vi "Top_Level.vi"() -> ()   [LabVIEW 2013]
uses:
  Classes/OSSP_Problem.lvclass
  Classes/GA.lvclass
  Classes/GA_Class/Controls/Solution.ctl
  Classes/GA_Class/Controls/Strategy.ctl
  Controls/States.ctl
  Classes/GA.lvclass/GA.ctl
  Classes/GA_Class/Evaluate Single Solution.vi
  Classes/GA_Class/Calculate Makespan.vi
  Classes/GA_Class/Select Random Solutions_2.vi
  Classes/GA_Class/One Point Crossover.vi
  Classes/Find Best Solution In Population.vi
  Classes/GA_Class/GA_Operation_To_MachineJobTuple.vi
  Classes/GA_Class/Find Gaps On Particular Machine.vi
  Classes/GA_Class/GA_Check_Other_Machines.vi
  Classes/GA_Class/GA_Schedule_Job.vi
  Classes/GA_Class/GA_Find_Job_On_Other_Machines.vi
  Classes/GA_Class/Find Elements not On Other Child.vi
  <vilib>/Analysis/baseanly.llb/Mean.vi
  <vilib>/Analysis/baseanly.llb/Mean (DBL).vi
  <vilib>/Analysis/1siggen.llb/Riffle.vi
  <vilib>/Analysis/1siggen.llb/Riffle Array (I32).vi
  Classes/GA_Class/GA_Increment_NumberofJobsOn Machine_ByOne.vi
panel:
  in  "Strategy":T1
  in  "Number of Generations":i32=1000
  in  "Population Size":u8=80
  in  "Mutation Probability":dbl=0.2
  in  "Crossover Probability":dbl=0.75
  out "Picture":picture
  out "Best Solution":T2
  out "GA.lvclass":refnum<class "GA.lvclass">
  out "OSSP_Problem.lvclass":refnum<class "OSSP_Problem.lvclass">
  out "error out":errorcluster
  in  "error in":errorcluster
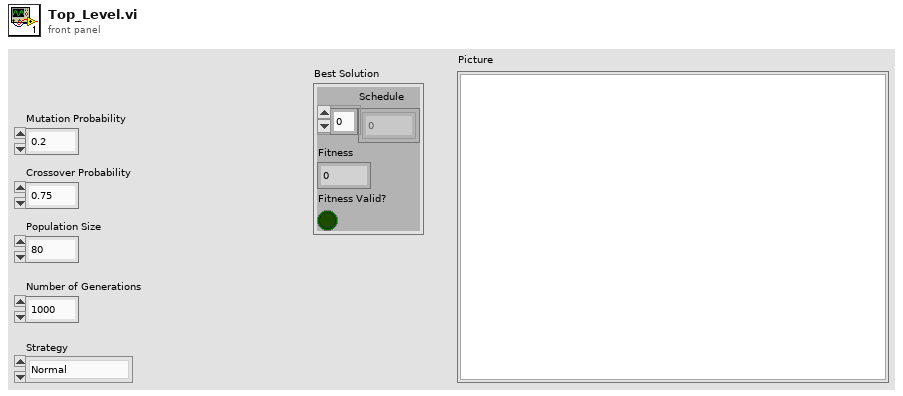
[diagram p1: front panel]
types:
  T1 = typedef "Strategy.ctl" = enum16{"Normal", "Ellitist 1", "Elitist 2"}
  T2 = typedef "Solution.ctl" = cluster{"Schedule":u16[], "Fitness":u16, "Fitness Valid?":bool}
  T3 = typedef "States.ctl" = enum16{"Read Problem", "Sort Problem", "Set Parameters", "Generate Initial Population", "Evaluate Initial Population", "Selection", "Crossover", "Mutation", "Evaluate New Population", "Replace Population with Offspring", "Record Best Solution", "Increment Population Counter", "Show Best Solution", "Plot", "Stop"}
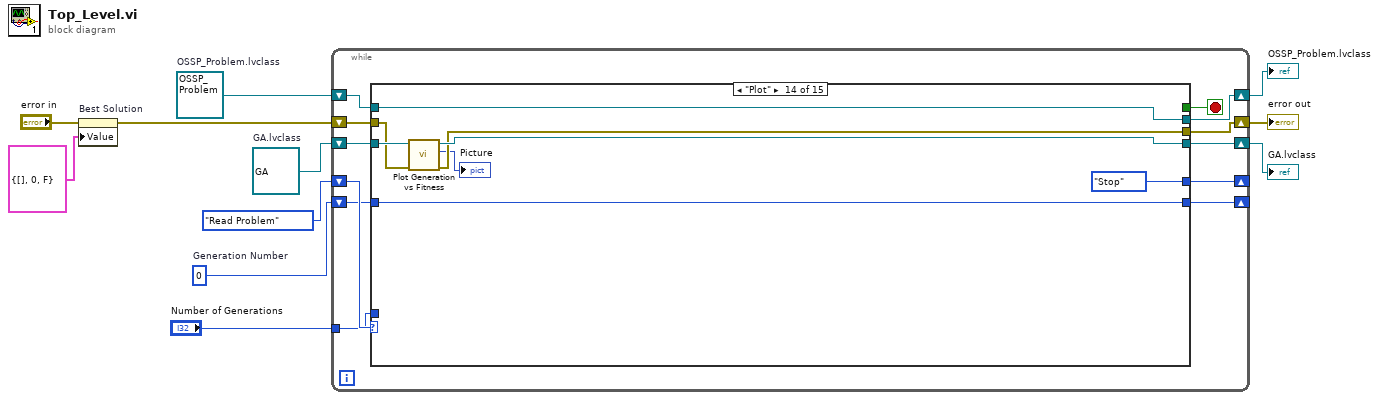
[diagram p0: block diagram]
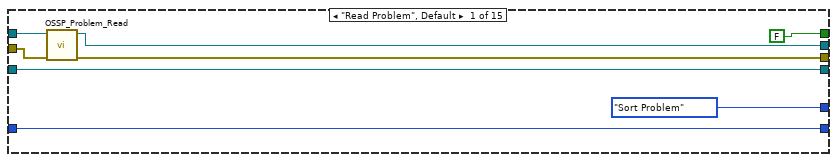
[diagram p2: hidden frame]
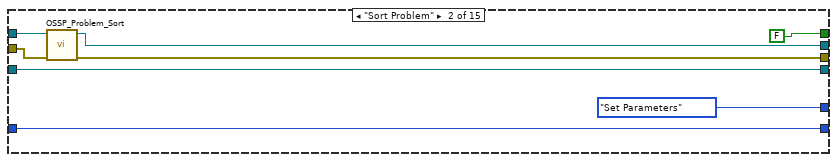
[diagram p3: hidden frame]
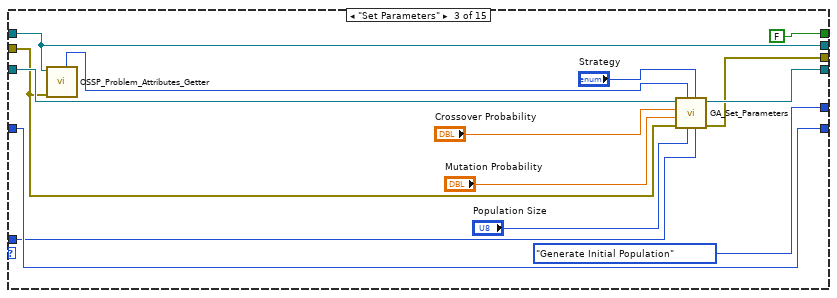
[diagram p4: hidden frame]
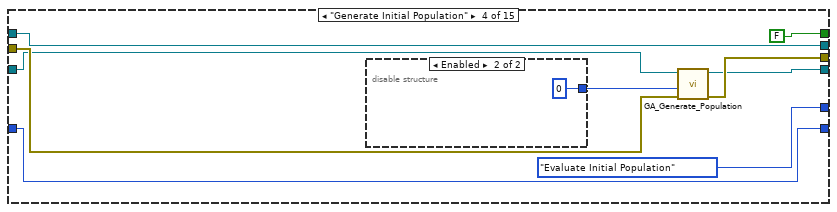
[diagram p5: hidden frame]
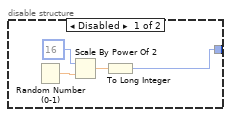
[diagram p6: hidden frame]
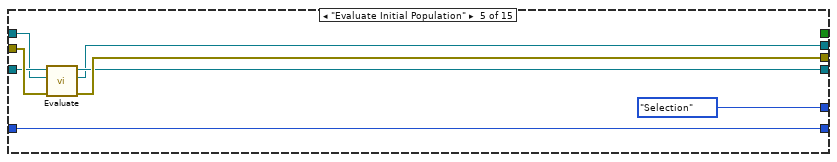
[diagram p7: hidden frame]
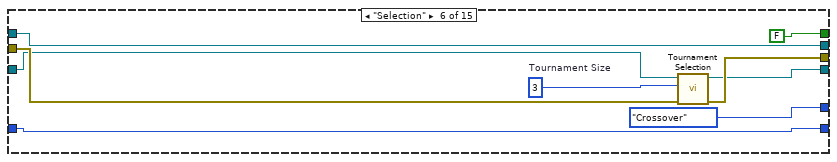
[diagram p8: hidden frame]
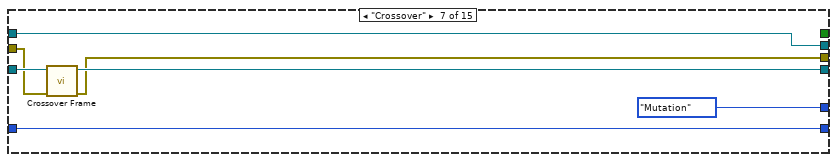
[diagram p9: hidden frame]
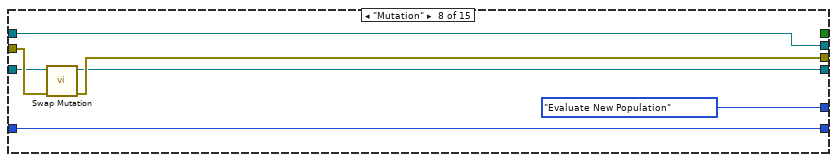
[diagram p10: hidden frame]
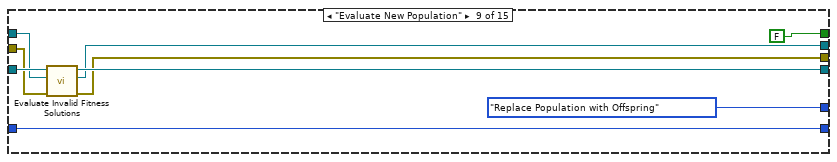
[diagram p11: hidden frame]
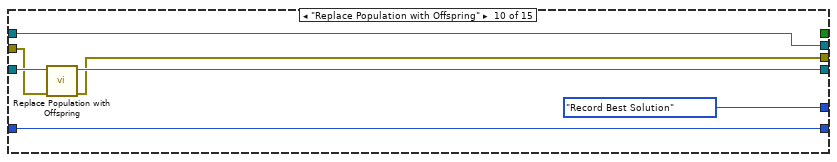
[diagram p12: hidden frame]
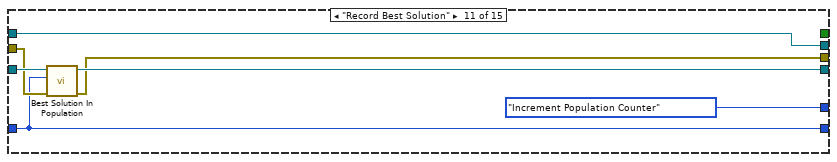
[diagram p13: hidden frame]
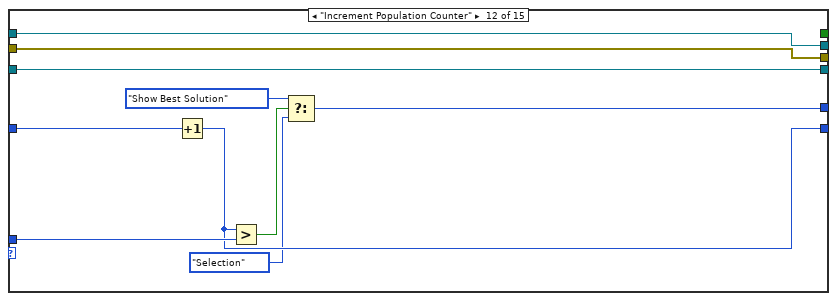
[diagram p14: hidden frame]
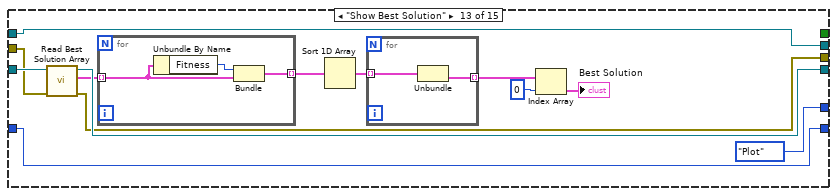
[diagram p15: hidden frame]
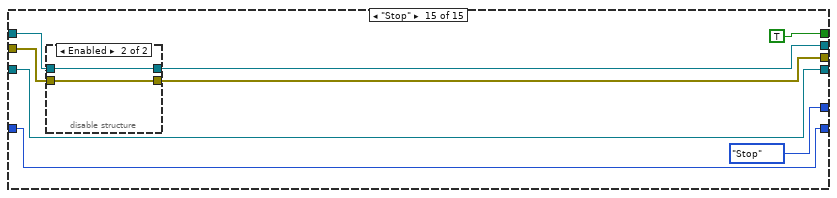
[diagram p16: hidden frame]
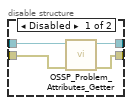
[diagram p17: hidden frame]
diagram:
  w5 = 0  # Generation Number
  w7 = refnum<class "GA.lvclass"> refnum  # GA.lvclass
  w9 = refnum<class "OSSP_Problem.lvclass"> refnum  # OSSP_Problem.lvclass
  n1 = property on="Best Solution" class="Clust (strict)"(error in="error in", "Value"=T2 {"Schedule"=[], "Fitness"=0, "Fitness Valid?"=FALSE} ("Best Solution")) -> (error out=w2:errorcluster)  [unwired: 1 in, 1 out]
  n2 = while {
    shift-right: [w21] -> _
    shift-left: States."Read Problem" -> [w23]
    shift-right: [w19] -> w10
    shift-left: w2 -> [w20]
    shift-right: [w17] -> w8
    shift-left: w9 -> [w18]
    shift-right: [w15] -> w4
    shift-left: w7 -> [w16]
    tunnel: "Number of Generations" -> [w14]
    shift-right: [w12] -> _
    shift-left: w5 -> [w13]
    stop <- w22 stop-if-true
    n3 = case shown="\"Plot\"" w23 {
      tunnel: [FALSE FALSE FALSE FALSE _ FALSE _ _ FALSE _ _ _ _ _ TRUE] -> w22
      tunnel: [States."Sort Problem" States."Set Parameters" States."Generate Initial Population" States."Evaluate Initial Population" States."Selection" States."Crossover" States."Mutation" States."Evaluate New Population" States."Replace Population with Offspring" States."Record Best Solution" States."Increment Population Counter" w123 States."Plot" States."Stop" States."Stop"] -> w21
      tunnel: w20 -> [w28 w37 w44 w59 w74 w78 w86 w95 w103 w109 w117 w131 w139 w152 w161]
      tunnel: [w27 w36 w47 w58 w73 w81 w85 w94 w102 w108 w116 w131 w138 w151 w160] -> w19
      tunnel: w18 -> [w29 w39 w45 w62 w70 w84 w91 w98 w101 w114 w121 w130 w144 w157 w163]
      tunnel: [w26 w38 w45 w62 w69 w84 w91 w98 w100 w114 w121 w130 w144 w157 w162] -> w17
      tunnel: w16 -> [w25 w33 w53 w57 w72 w77 w88 w93 w105 w111 w119 w129 w141 w154 w159]
      tunnel: [w25 w33 w50 w56 w71 w76 w87 w92 w104 w110 w118 w129 w140 w153 w159] -> w15
      tunnel: w14 -> [_ _ w41 _ _ _ _ _ _ _ _ w127 _ _ _]
      tunnel: [w24 w32 w42 w55 w68 w82 w89 w97 w107 w113 w115 w125 w143 w156 w158] -> w12
      tunnel: w13 -> [w24 w32 w42 w55 w68 w82 w89 w97 w107 w113 w115 w128 w143 w156 w158]
      frame "Read Problem", Default {
        n4 = call "OSSP_Problem_Read.vi"("error in (no error)"=w28, "OSSP_Problem.lvclass In"=w29) -> ("error out"=w27:errorcluster, "OSSP_Problem.lvclass Out"=w26:refnum<class "OSSP_Problem.lvclass">)  [unwired: 8 in]
      }
      frame "Sort Problem" {
        n5 = call "OSSP_Problem_Sort.vi"("error in (no error)"=w37, "OSSP_Problem.lvclass In"=w39) -> ("error out"=w36:errorcluster, "OSSP_Problem.lvclass Out"=w38:refnum<class "OSSP_Problem.lvclass">)  [unwired: 8 in]
      }
      frame "Set Parameters" {
        n6 = call "OSSP_Problem_Attributes_Getter.vi"("error in (no error)"=w44, "OSSP_Problem in"=w45) -> ("Dimension"=w43:i32)  [unwired: 4 in, 5 out]
        n7 = call "GA_Set_Parameters.vi"("Number of Generations"=w41, "Strategy"="Strategy", "Population Size"="Population Size", "Dimension"=w43, "error in (no error)"=w44, "Control 1Mutation Probability"="Mutation Probability", "Crossover Probability"="Crossover Probability", "GA in"=w53) -> ("error out"=w47:errorcluster, "GA out"=w50:refnum<class "GA.lvclass">)  [unwired: 2 in]
      }
      frame "Generate Initial Population" {
        n8 = disable-structure shown="Enabled" {
          disable-tunnel: [w63 0 ("seed")] -> w54
          frame Disabled {
            n9 = Random Number (0-1)() -> (number: 0 to 1=w65:dbl)
            n10 = Scale By Power Of 2(n=16, x=w65) -> (x*2^n=w64:dbl)
            n11 = To Long Integer(number=w64) -> (32bit integer=w63:i32)
          }
          frame Enabled {
          }
        }
        n12 = call "GA_Generate_Population.vi"("error in (no error)"=w59, "seed"=w54, "GA in"=w57) -> ("error out"=w58:errorcluster, "GA out"=w56:refnum<class "GA.lvclass">)  [unwired: 7 in]
      }
      frame "Evaluate Initial Population" {
        n13 = call "Evaluate.vi"("error in (no error)"=w74, "OSSP_Problem.lvclass"=w70, "GA in"=w72) -> ("error out"=w73:errorcluster, "OSSP_Problem out"=w69:refnum<class "OSSP_Problem.lvclass">, "GA out"=w71:refnum<class "GA.lvclass">)  [unwired: 6 in]
      }
      frame "Selection" {
        w80 = 3  # Tournament Size
        n14 = call "Tournament Selection.vi"("error in (no error)"=w78, "Tournament Size"=w80, "GA.lvclass In"=w77) -> ("error out"=w81:errorcluster, "GA.lvclass Out"=w76:refnum<class "GA.lvclass">)  [unwired: 7 in]
      }
      frame "Crossover" {
        n15 = call "Crossover Frame.vi"("error in (no error)"=w86, "GA in"=w88) -> ("error out"=w85:errorcluster, "GA out"=w87:refnum<class "GA.lvclass">)  [unwired: 8 in]
      }
      frame "Mutation" {
        n16 = call "Swap Mutation.vi"("error in (no error)"=w95, "GA in"=w93) -> ("error out"=w94:errorcluster, "GA out"=w92:refnum<class "GA.lvclass">)  [unwired: 8 in]
      }
      frame "Evaluate New Population" {
        n17 = call "Evaluate Invalid Fitness Solutions.vi"("error in (no error)"=w103, "OSSP_Problem.lvclass"=w101, "GA in"=w105) -> ("error out"=w102:errorcluster, "OSSP_Problem out"=w100:refnum<class "OSSP_Problem.lvclass">, "GA out"=w104:refnum<class "GA.lvclass">)  [unwired: 6 in]
      }
      frame "Replace Population with Offspring" {
        n18 = call "Replace Population with Offspring.vi"("error in (no error)"=w109, "GA in"=w111) -> ("error out"=w108:errorcluster, "GA out"=w110:refnum<class "GA.lvclass">)  [unwired: 8 in]
      }
      frame "Record Best Solution" {
        n19 = call "Best Solution In Population.vi"("error in (no error)"=w117, "Generation Number"=w115, "GA in"=w119) -> ("error out"=w116:errorcluster, "GA out"=w118:refnum<class "GA.lvclass">)  [unwired: 7 in]
      }
      frame "Increment Population Counter" {
        n20 = Increment(x=w128) -> (x+1=w125:i32)
        n21 = Greater?(x=w125, y=w127) -> (0:w126:bool)
        n22 = Select(t=States."Show Best Solution", s=w126, f=States."Selection") -> (s? t:f=w123:T3)
      }
      frame "Show Best Solution" {
        n23 = call-dynamic "Read Best Solution Array.vi"("error in (no error)"=w139, "GA in"=w141) -> ("error out"=w138:errorcluster, "Best Solution Array"=w137:T2[], "GA out"=w140:refnum<class "GA.lvclass">)  [unwired: 7 in]
        n24 = for {
          tunnel: w137 -> [w148] mode=indexing
          tunnel: [w147] -> w136 mode=indexing
          n25 = Unbundle By Name(w148) -> ("Fitness"=w149:u16)
          n26 = Bundle("Fitness"=w149, "Solution"=w148) -> (w147:cluster{"Fitness":u16, "Solution":T2})  [unwired: 1 in]
        }
        n27 = Sort 1D Array(array=w136) -> (sorted array=w135:cluster{"Fitness":u16, "Solution":T2}[])
        n28 = for {
          tunnel: w135 -> [w146] mode=indexing
          tunnel: [w145] -> w134 mode=indexing
          n29 = Unbundle(w146) -> ("Solution"=w145:T2)  [unwired: 1 out]
        }
        n30 = Index Array(array=w134, index=0) -> (element=→"Best Solution":T2)
      }
      frame "Plot" {
        n31 = call "Plot Generation vs Fitness.vi"("error in (no error)"=w152, "GA in"=w154) -> ("error out"=w151:errorcluster, "Picture"=→"Picture":picture, "GA out"=w153:refnum<class "GA.lvclass">)  [unwired: 7 in]
      }
      frame "Stop" {
        n32 = disable-structure shown="Enabled" {
          disable-tunnel: w163 -> [w169 w171]
          disable-tunnel: [w168 w171] -> w162
          disable-tunnel: w161 -> [w167 w170]
          disable-tunnel: [w166 w170] -> w160
          frame Disabled {
            n33 = call "OSSP_Problem_Attributes_Getter.vi"("error in (no error)"=w167, "OSSP_Problem in"=w169) -> ("error out"=w166:errorcluster, "OSSP_Problem out"=w168:refnum<class "OSSP_Problem.lvclass">)  [unwired: 4 in, 4 out]
          }
          frame Enabled {
          }
        }
      }
    }
  }
  "error out" <- w10
  "OSSP_Problem.lvclass" <- w8
  "GA.lvclass" <- w4
